vi "NLEIS_Run_PXI.vi"(0 "# of Amplitudes\n(Auto)":i32=5, 1 "Largest Amplitude (mA or mV)":dbl=0.01 format="%#.5f", 2 "Smallest Amplitude (mA or mV)":dbl=0.005 format="%#.6f", 4 "Steps/Decade":dbl=10.0, 5 "High Frequency (Hz)":dbl=10000.0, 6 "Internal Resistor":string(combo), 7 "Low Frequency (Hz)":dbl=1.0, 8 "Overload Action":string(combo)="OL0", 9 "File Path to Save":path=path "C:/Users/Giang/Desktop/NLEIS_test/test/1", 10 "Perturbation Input Gain":string(combo)="PI1", 11 "Amplitude Scaling File Location":path=path "C:/Users/Giang/Desktop/scaling_factors.txt", 12 "Voltage Output Gain":string(combo)="VX0", 14 "Current Output Gain":string(combo)="IX0") -> ()   [LabVIEW 2018]
doc: "This example shows the Standard Function output mode. \n\nIt also shows some of the parameters which can be changed on the fly."
uses:
  <vilib>/Utility/file.llb/Read From Spreadsheet File (DBL).vi
  <vilib>/Utility/file.llb/Write To Spreadsheet File (string).vi
panel:
  out "Error code 2":dbl
  out "Error code 1":dbl caption="Potentiostat \nError code 1"
  in  "Graph Tabs":enum32{"Active Run", "Nyquist Plot"}(tab)
  out "Avg Voltage FFT":cluster{"f0":dbl, "df":dbl, "magnitude":dbl[]}(graph)
  out "Avg Current FFT":cluster{"f0":dbl, "df":dbl, "magnitude":dbl[]}(graph)
  out "Avg I & V (Scaled)":waveform(dbl)[](graph) caption="Waveform \nGraph 3"
  in  "V Scale":dbl(slide) min=-6.0 max=0.0 step=1.0 scale=0.0..-6.0
  in  "I Scale":dbl(slide)=-3.0 min=-6.0 max=0.0 step=1.0 scale=0.0..-6.0
  out "Nyquist Plot":cluster{"Y":dbl[], "Y":dbl[]}[](graph)
  out "Actual End Time":timestamp format="%<%I:%M:%S %p\n%x>T"
  in  "NLEIS Run Mode":bool caption="Test        Sweep"
  in  "Bottom Tabs":enum32{"Status", "Generated Arrays"}(tab)
  out "Estimated End Time":timestamp format="%<%I:%M:%S %p\n%x>T"
  out "# Freqs":i32
  out "Actual Frequency":dbl format="%.6f"
  out "Freq Index":i32
  out "IR In Use":string
  out "FGEN Amp (V)":dbl
  out "Digitizer Loop\nComplete":bool
  out "Amp Index":i32
  out "# Amps":i32
  out "Cut-off Exceeded":bool
  out "Solartron Error":bool
  out "fp":dbl[](array[numeric]) format="%#.8f"
  out "Scaling Factors":sgl[](array[numeric])
  out "Amplitudes":dbl[](array[numeric])
  out "DAQ Error":string
  out "FGen Error":string caption="FGEN Error"
  out "DAQ Input":waveform(dbl)[](graph) caption="Waveform \nGraph 3"
  out "Pre-Check Voltage":dbl[](graph)
  in  "Middle Tabs":T1(tab)
  in  "Bandwidth":string(combo)="2"
  in  "Operation Mode":bool=TRUE
  in  "EIS File":bool
  in  "Time Files":bool=TRUE
  in  "Potentiostat":refnum<visa-resource-name>="Solartron1287"
  in  "FGen":refnum<k15>="FGEN-5421" caption="Waveform Generator"
  in  "NISCOPE":refnum<k15>="NISCOPE-5922" caption="Oscilloscope"
  in  "BiasReject ON?":bool
  in  "# Pre-Checks (>1Hz)":i32=10
  in  "Fixed Voltage Rejection (VRF)":string="VR0"
  in  "Fixed Current Rejection (IRF)":string="IR0"
  in  "Pre-Check Cut-Off (V)":dbl=0.5
  in  "# Pre-Checks (<1Hz)":i32=1
  in  "Direct Bias":string="PC0" caption="PCF (Amps)\nPVF (Volts)"
  in  "Bias Reject Mode":bool
  in  "Channel 1 (Voltage)":dbl=2.0
  in  "Channel 0 (Current)":dbl=2.0
  in  "Top Tabs":enum32{"Test", "Sweep", "Adv. Setup"}(tab)
  in  "Test Amplitude (mA or mV)":dbl=0.005
  in  "Peak Frequency (Hz)":dbl=5.0
  out "Too Many?":bool
  in  "Sweep Direction":bool
  in  "Crossover Freqs":string
  in  "Variable Resistor":bool
  in  "Manual # of Averages":i32=1
  in  "Signal Averages Selection":bool
  in  "# of Amps\n(Manual)":i32
  in  "Amplitude\nArray Source":bool
  in  "Manual Amplitudes":dbl[](array[numeric])
  # "Raw Digitizer Inputs"
  # "Pre-Check Voltage (Potentiostat)"
  # "Average Current and Voltage"
  # "Average Current Harmonics (FFT)"
  # "Average Voltage Harmonics (FFT)"
  # "Sweep Details"
  # "Active Run"
  # "Electrochemical Interface (SI1287) Setup"
  # "Write Files"
  # "Electrochemical Interface (SI1287) Setup"
  # "Bias Settings"
  # "Signal Precheck"
  # "Electrochemical Interface (SI1287) Setup"
  # "PStat Gain Control"
  # "PXI-5922 has two vertical range: \n1) 2 Vpk-pk, -1 -> +1 V\n2) 10 vpk-pk, -5 -> +5V"
  # "Vertical Range"
  # "Harmonic Tests Setup"
  # "Frequency Sweep Setup"
  # "Perturbation Amplitude Sweep (Auto)"
  # "Signal Processing Averaging Setup"
  # "Perturbation Amplitude Sweep (Manual)"
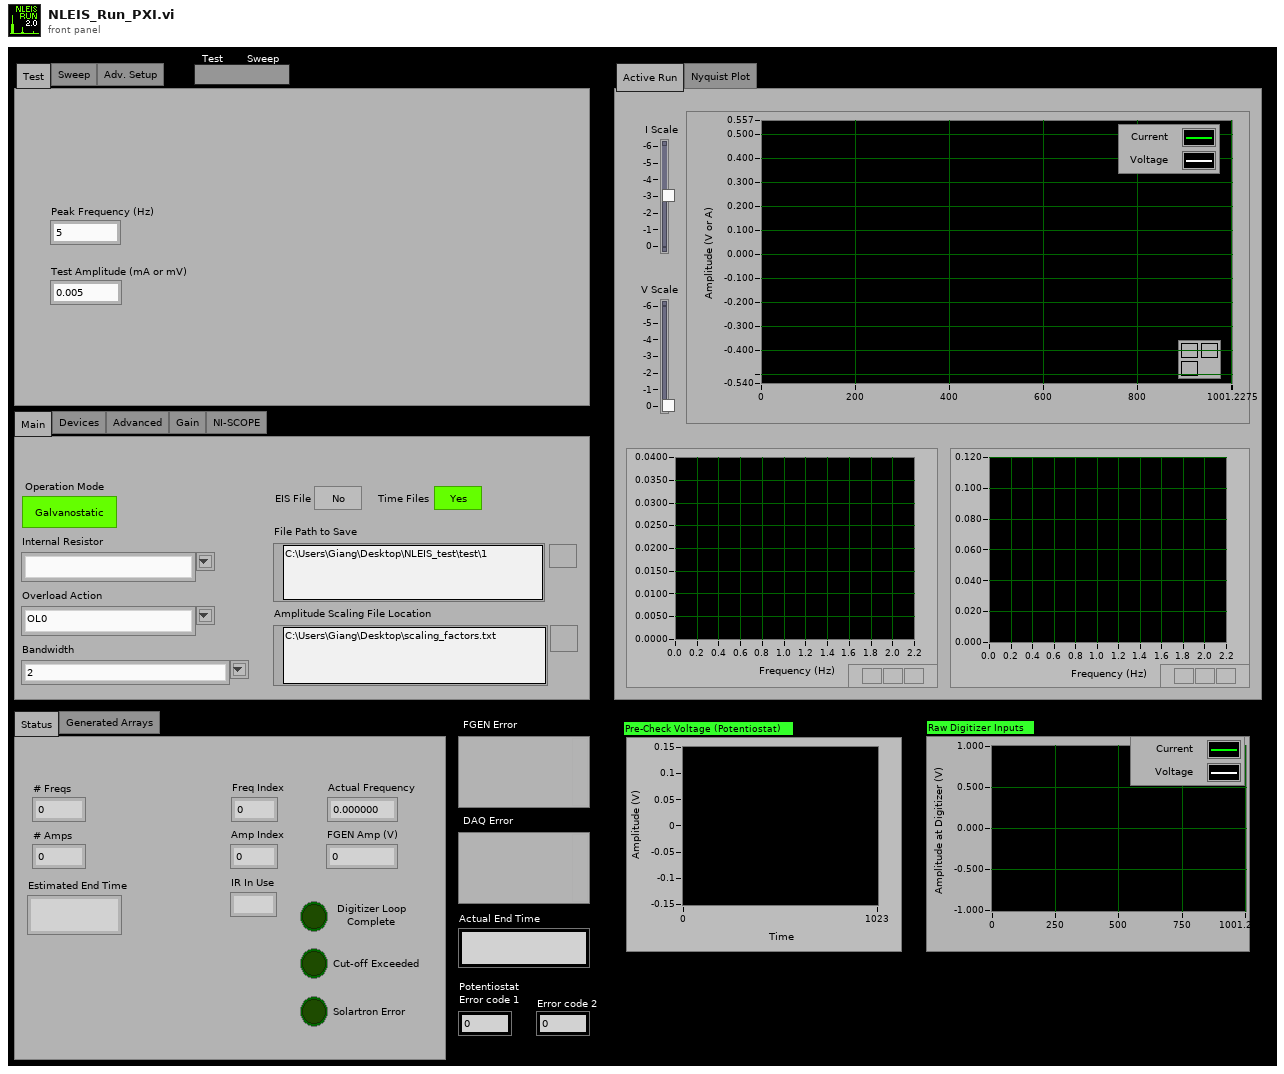
[diagram p1: front panel]
types:
  T1 = enum32{"Main", "Devices", "Advanced", "Gain", "NI-SCOPE"}
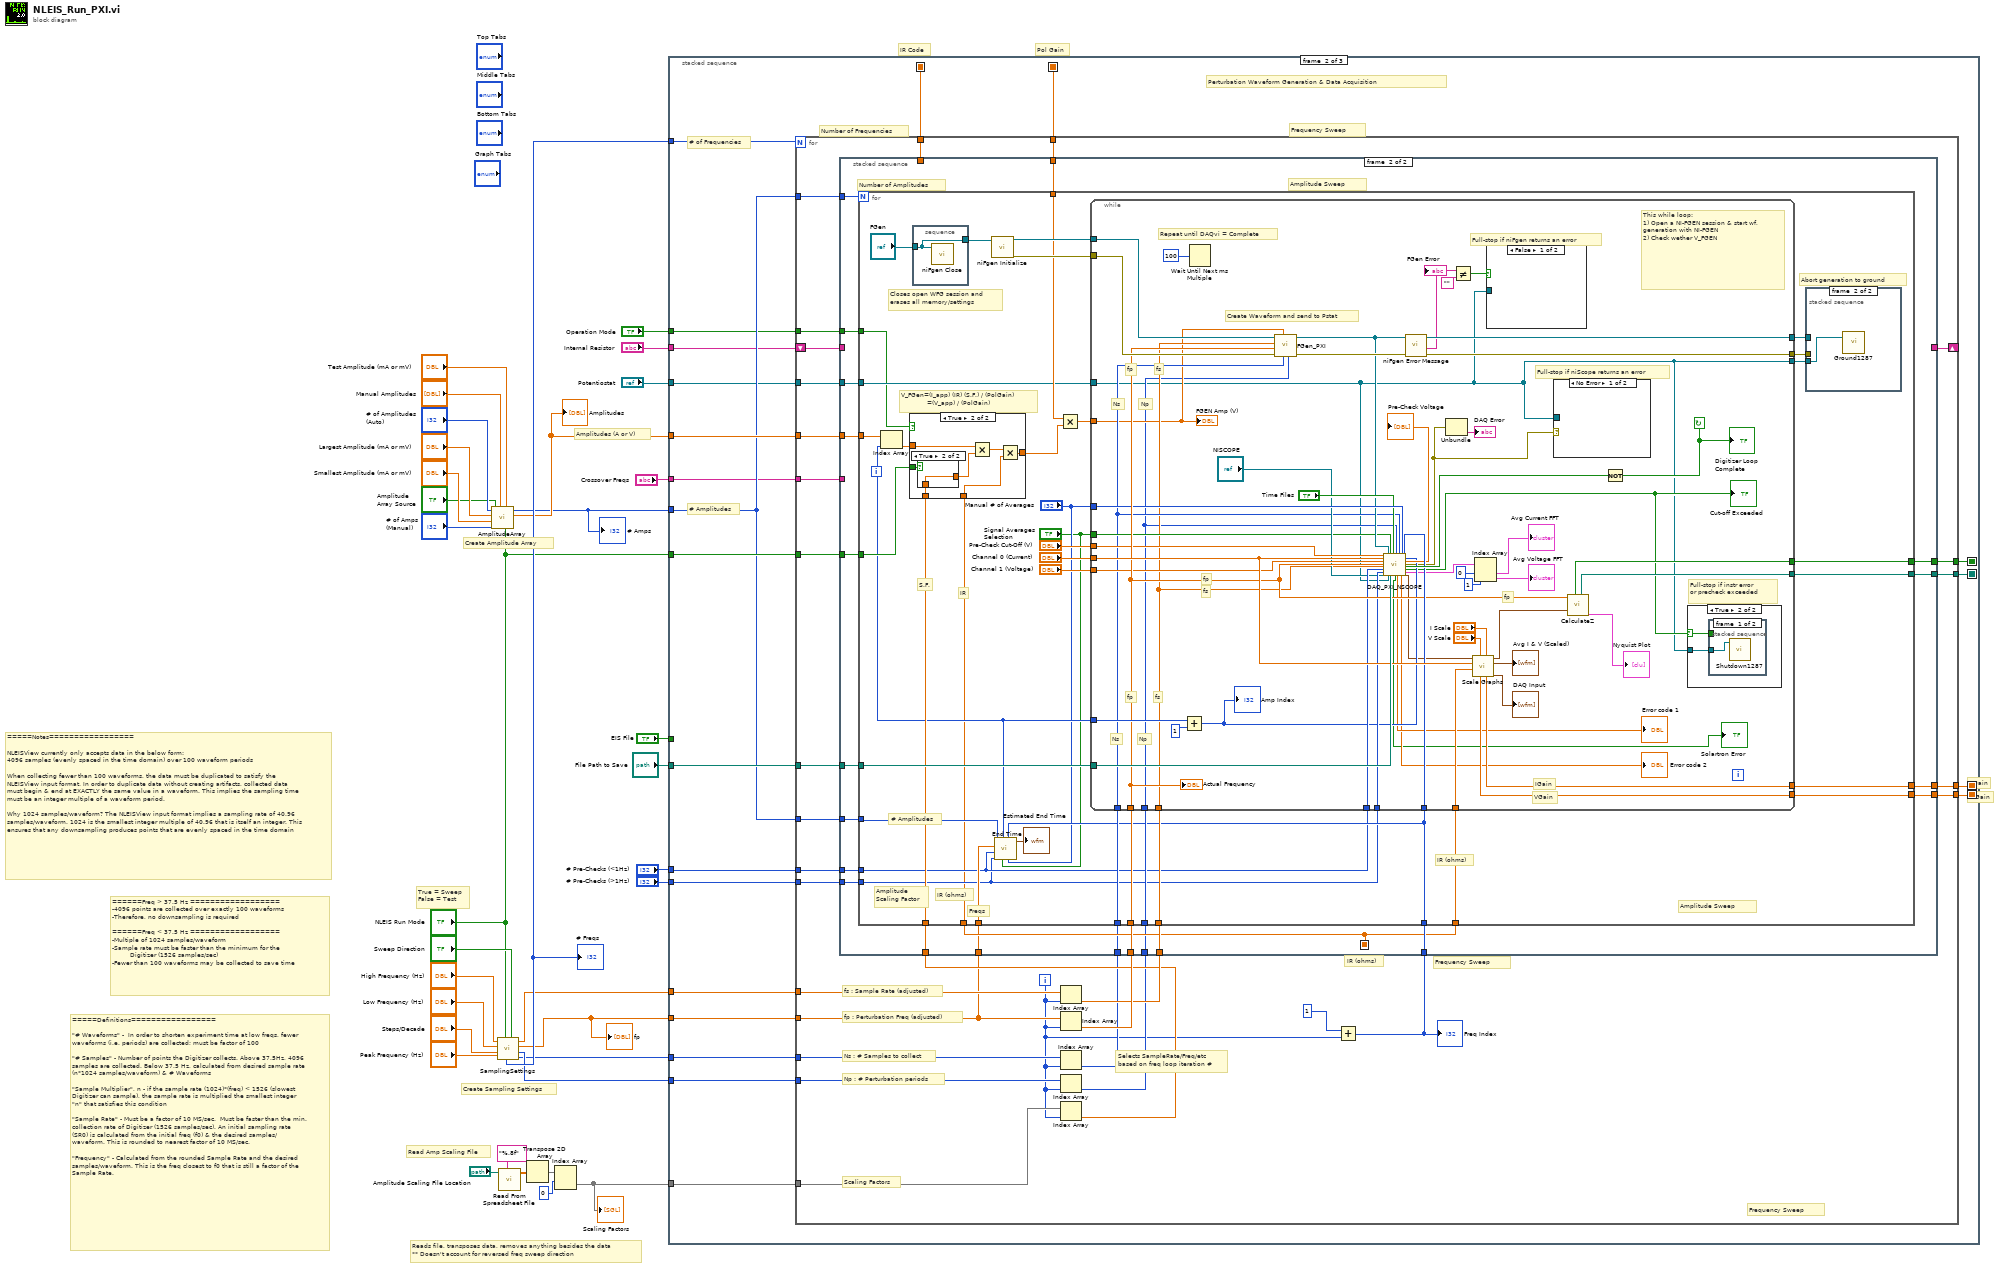
[diagram p0: block diagram]
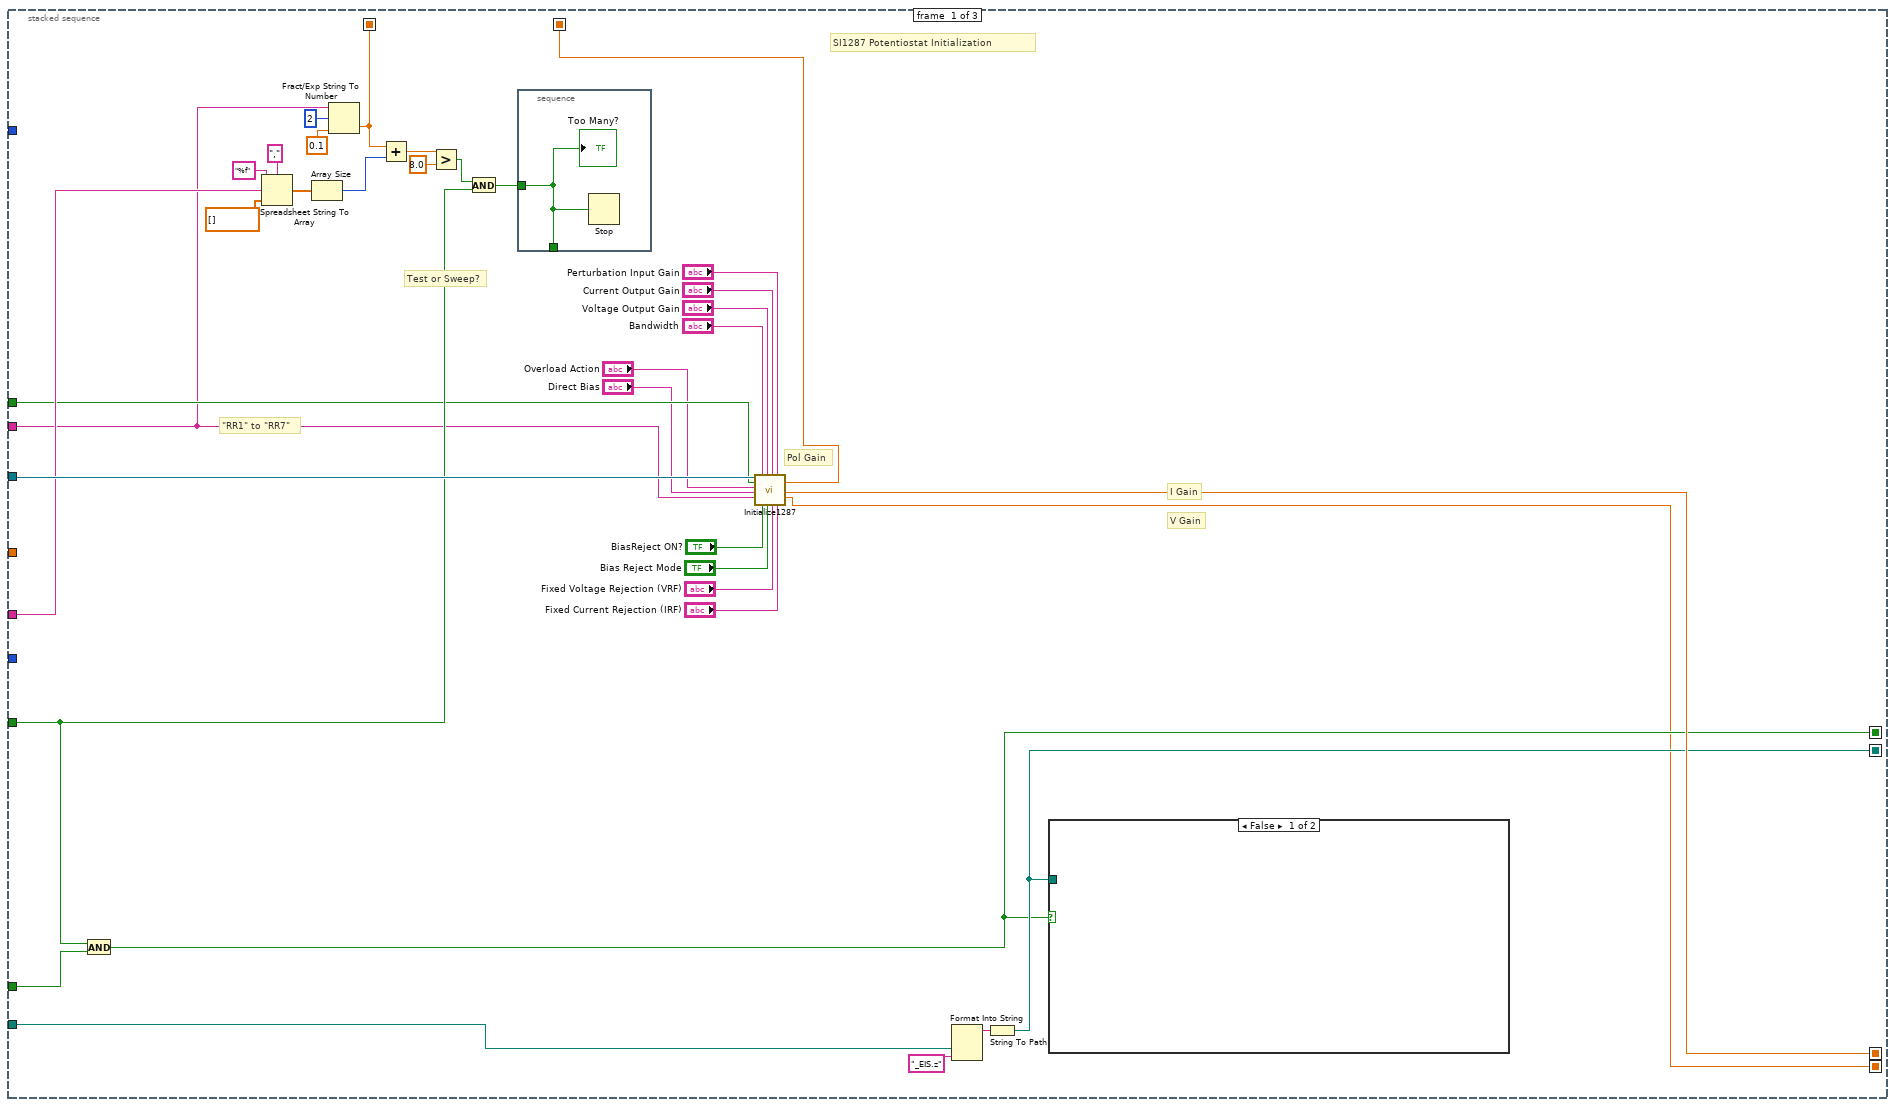
[diagram p2: hidden frame]
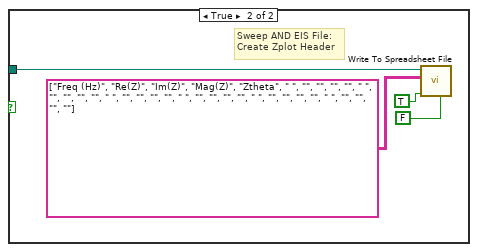
[diagram p3: hidden frame]
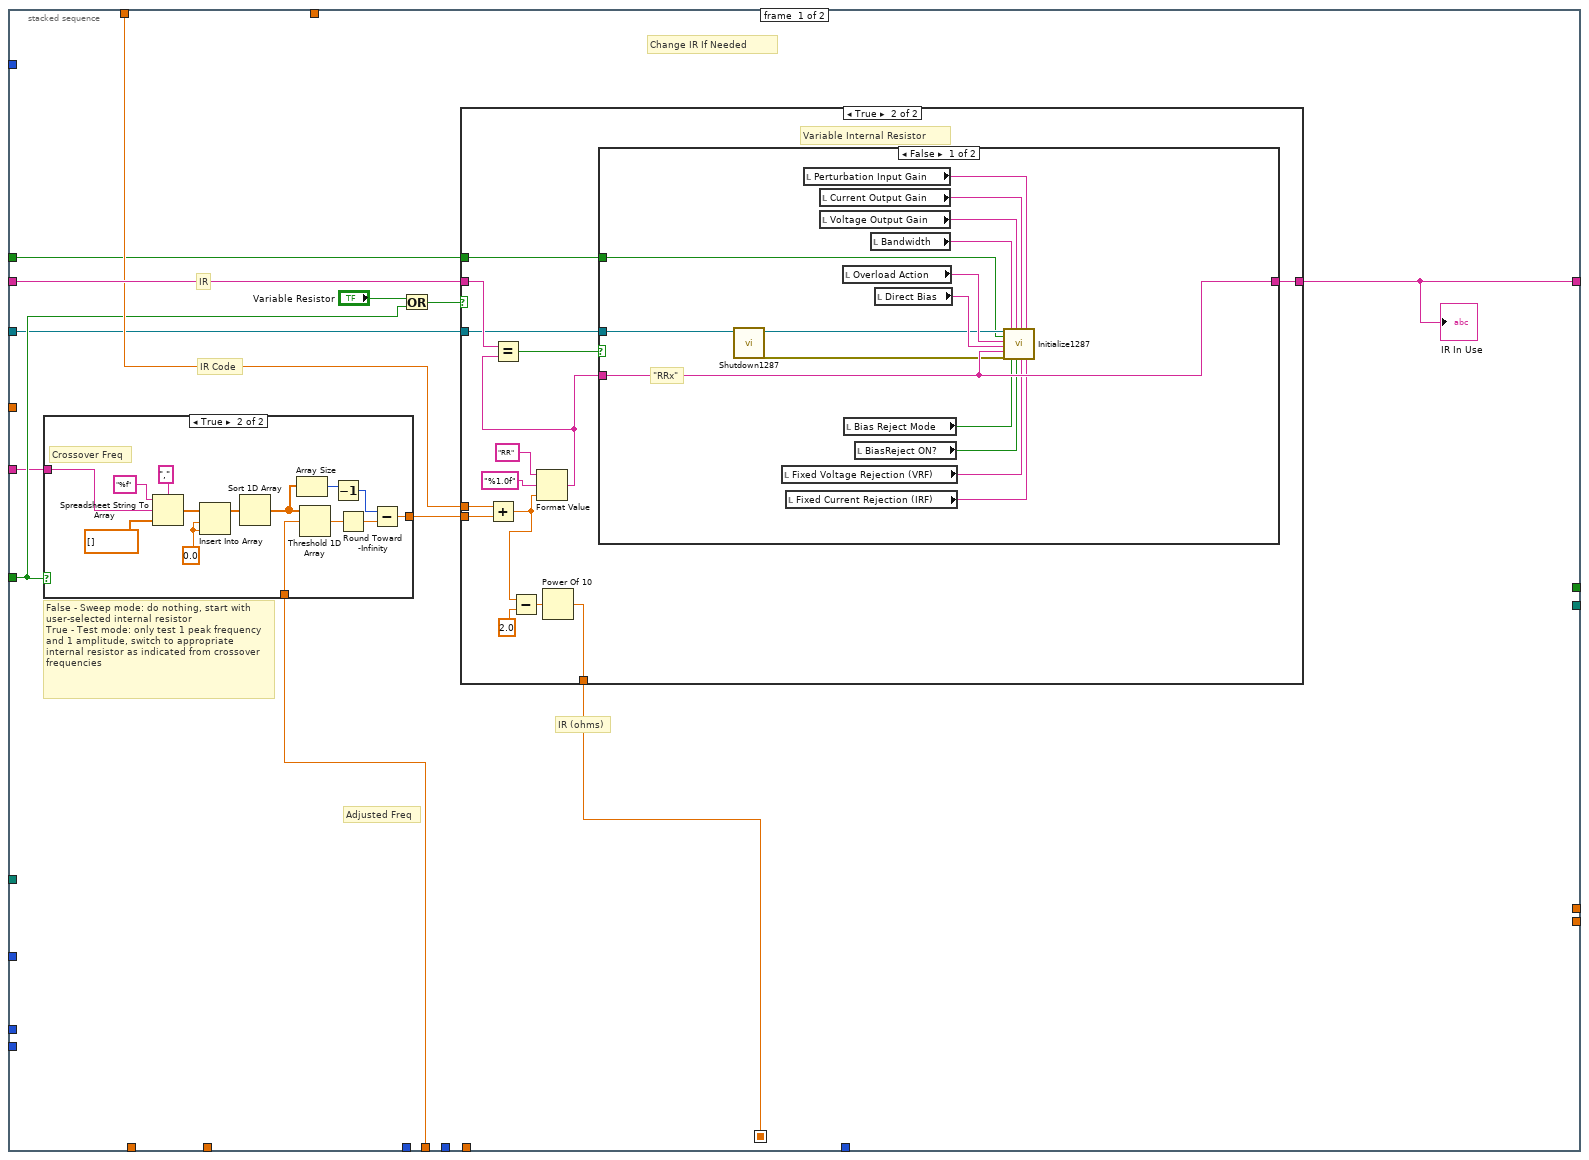
[diagram p4: hidden frame]
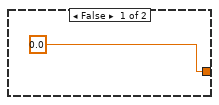
[diagram p5: hidden frame]
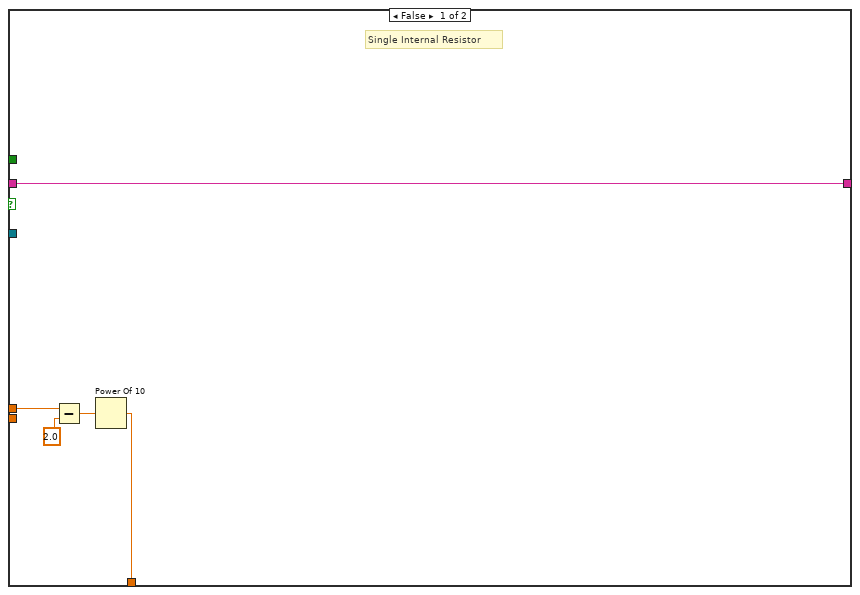
[diagram p6: hidden frame]
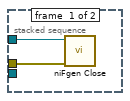
[diagram p8: hidden frame]
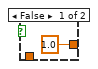
[diagram p10: hidden frame]
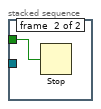
[diagram p12: hidden frame]
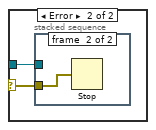
[diagram p13: hidden frame]
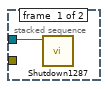
[diagram p14: hidden frame]
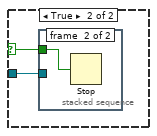
[diagram p15: hidden frame]
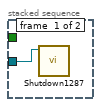
[diagram p16: hidden frame]
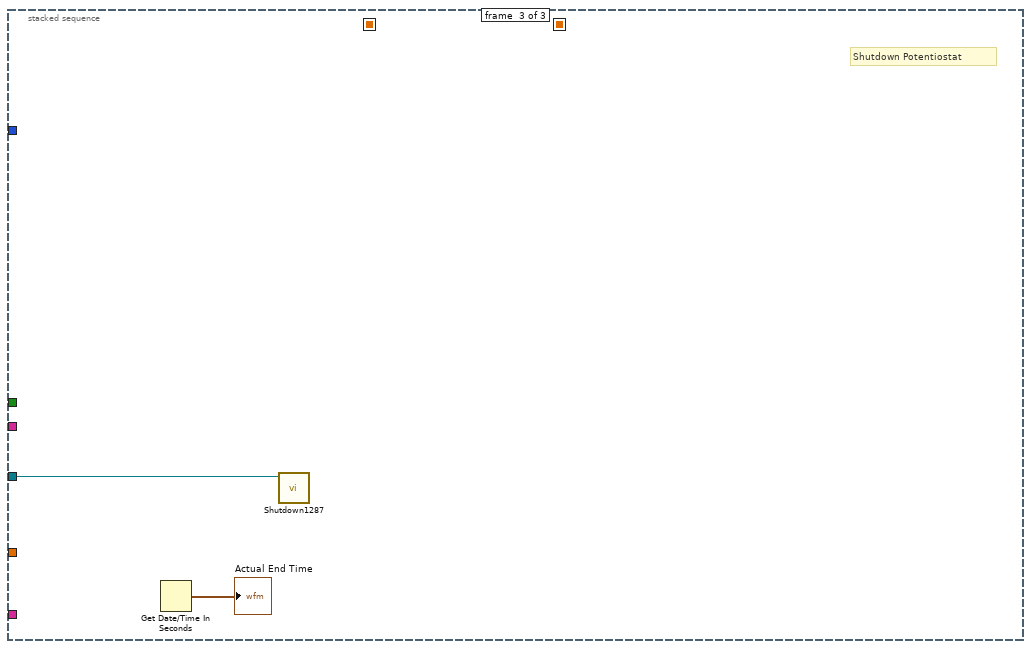
[diagram p17: hidden frame]
diagram:
  # "Amplitudes (A or V)"
  # "True = Sweep\nFalse = Test"
  # "Read Amp Scaling File"
  # "Reads file, transposes data, removes anything besides the data\n** Doesn't account for reversed freq sweep direction"
  # "V Gain"
  # "I Gain"
  # "IR Code"
  # "Pol Gain"
  # "Create Sampling Settings"
  # "Create Amplitude Array"
  # "=====Notes=================\n\nNLEISView currently only accepts data in the below form:\n4096 samples (evenly spaced in the time domain) over 100 waveform periods\n\nWhen collecting fewer than 100 waveforms, the data must be duplicated to satisfy the NLEISView input format. In order to duplicate data without creating artifacts, collected data must begin & end at EXACTLY the same value in a waveform. This implies the sampling time must be an integer multiple of a waveform period.\n\nWhy 1024 samples/waveform? The NLEISView input format implies a sampling rate of 40.96 samples/waveform. 1024 is the smallest integer multiple of 40.96 that is itself an integer. This ensures that any downsampling produces points that are evenly spaced in the time domain"
  # "=====Definitions=================\n\n\"# Waveforms\" -  In order to shorten experiment time at low freqs, fewer waveforms (i.e. periods) are collected; must be factor of 100\n\n\"# Samples\" - Number of points the Digitizer collects. Above 37.5Hz, 4096 samples are collected. Below 37.5 Hz, calculated from desired sample rate (n*1024 samples/waveform) & # Waveforms\n\n\"Sample Multiplier\", n - if the sample rate (1024)*(freq) < 1526 (slowest Digitizer can sample), the sample rate is multiplied the smallest integer \"n\" that satisfies this condition\n\n\"Sample Rate\" - Must be a factor of 10 MS/sec.  Must be faster than the min. collection rate of Digitizer (1526 samples/sec). An initial sampling rate (SR0) is calculated from the initial freq (f0) & the desired samples/waveform. This is rounded to nearest factor of 10 MS/sec.\n\n\"Frequency\" - Calculated from the rounded Sample Rate and the desired samples/waveform. This is the freq closest to f0 that is still a factor of the Sample Rate."
  # "======Freq > 37.5 Hz ==================\n-4096 points are collected over exactly 100 waveforms\n-Therefore, no downsampling is required\n\n======Freq < 37.5 Hz ==================\n-Multiple of 1024 samples/waveform\n-Sample rate must be faster than the minimum for the \n         Digitizer (1526 samples/sec)\n-Fewer than 100 waveforms may be collected to save time"
  n1 = call "AmplitudeArray.vi"("NLEIS Run Mode"="NLEIS Run Mode", "Test Amplitude (mA)"="Test Amplitude (mA or mV)", "Amplitude\nArray Source"="Amplitude\nArray Source", "Manual Amplitudes"="Manual Amplitudes", "# Amplitudes (Manual)"="# of Amps\n(Manual)", "Smallest Amplitude (mA)"="Smallest Amplitude (mA or mV)", "Largest Amplitude (mA)"="Largest Amplitude (mA or mV)", "# Amplitudes (Auto)"="# of Amplitudes\n(Auto)") -> ("Amplitudes (A)"=w17:dbl[], "# Amplitudes"=w4:i32)  [unwired: 2 in]
  "Amplitudes" <- w17
  "# Amps" <- w4
  n2 = call "SamplingSettings.vi"("Sweep Direction"="Sweep Direction", "NLEIS Run Mode"="NLEIS Run Mode", "Peak Frequency (Hz)"="Peak Frequency (Hz)", "Steps/Decade"="Steps/Decade", "Low Frequency (Hz)"="Low Frequency (Hz)", "High Frequency (Hz)"="High Frequency (Hz)") -> ("N Samples"=w25:i32[], "Np Periods"=w26:i32[], "Freqs"=w9:dbl[], "Sample Rates"=w27:dbl[], "Number of Frequencies"=w28:i32)  [unwired: 1 out]
  "# Freqs" <- w28
  "fp" <- w9
  n3 = call-poly <vilib>:"Read From Spreadsheet File.vi"("format (%.3f)"="%.8f", "file path (dialog if empty)"="Amplitude Scaling File Location") -> ("all rows"=w12:dbl[][])  [unwired: 5 in, 4 out]
  n4 = Transpose 2D Array(2D array=w12) -> (transposed array=w11:dbl[][])
  n5 = Index Array(array=w11, index (row)=0) -> (element=w10:dbl[])  [unwired: 1 in]
  "Scaling Factors" <- w10
  n6 = stacked-sequence {
    seq-local: [w62 _ _] -> [_ w93 _]
    seq-local: [w36 _ _] -> [_ w92 _]
    seq-local: [w35 _ _] -> [_ w91 _]
    seq-local: [w57 _ _] -> [_ w90 _]
    seq-local: [w52 _ _] -> [_ w79 _]
    seq-local: [w49 _ _] -> [_ w78 _]
    tunnel: "File Path to Save" -> [w53 w97 _]
    tunnel: w28 -> [_ w96 _]
    tunnel: w9 -> [_ w95 _]
    tunnel: w27 -> [_ w94 _]
    tunnel: "NLEIS Run Mode" -> [w50 w87 _]
    tunnel: w25 -> [_ w89 _]
    tunnel: w26 -> [_ w88 _]
    tunnel: w17 -> [_ w86 _]
    tunnel: w4 -> [_ w85 _]
    tunnel: w10 -> [_ w84 _]
    tunnel: "# Pre-Checks (<1Hz)" -> [_ w83 _]
    tunnel: "# Pre-Checks (>1Hz)" -> [_ w82 _]
    tunnel: "Potentiostat" -> [w58 w81 w334]
    tunnel: "Crossover Freqs" -> [w56 w80 _]
    tunnel: "EIS File" -> [w51 _ _]
    tunnel: "Operation Mode" -> [w44 w76 _]
    tunnel: "Internal Resistor" -> [w41 w77 _]
    frame #0 {
      # "\"RR1\" to \"RR7\""
      # "I Gain"
      # "V Gain"
      # "Pol Gain"
      # "Test or Sweep?"
      # "SI1287 Potentiostat Initialization"
      n7 = And(x=w50, y=w51) -> (x .and. y?=w49:bool)
      n8 = Spreadsheet String To Array(delimiter (Tab)=",", format string="%f", spreadsheet string=w56, array type (2D Dbl)=dbl[] []) -> (array=w61:dbl[])
      n9 = Array Size(array=w61) -> (size(s)=w65:i32)
      n10 = Fract/Exp String To Number(string=w41, offset=2, default (0 dbl)=0.1) -> (number=w62:dbl)  [unwired: 1 in, 1 out]
      n11 = Add(x=w62, y=w65) -> (x+y=w64:dbl)
      n12 = Greater?(x=w64, y=8.0) -> (0:w60:bool)
      n13 = And(x=w60, y=w50) -> (x .and. y?=w59:bool)
      n14 = stacked-sequence {
        tunnel: [w75] -> _
        tunnel: w59 -> [w75]
        frame #0 {
          n15 = Stop(stop? (T)=w75) -> ()
          "Too Many?" <- w75
        }
      }
      n16 = call "Initialize1287.vi"("VISA Name In"=w58, "Operation Mode"=w44, "Overload Action"="Overload Action", "DC Bias"="Direct Bias", "Internal Resistor"=w41, "Bandwidth"="Bandwidth", "Bias Rejection ON?"="BiasReject ON?", "Voltage Gain"="Voltage Output Gain", "Bias Reject Mode"="Bias Reject Mode", "Current Gain"="Current Output Gain", "Fixed Voltage Rejection"="Fixed Voltage Rejection (VRF)", "Perturbation Waveform Gain"="Perturbation Input Gain", "Fixed Current Rejection"="Fixed Current Rejection (IRF)") -> ("Pol Gain Correction"=w36:dbl, "I Gain Correction"=w57:dbl, "V Gain Correction"=w35:dbl)  [unwired: 2 in, 2 out]
      n17 = Format Into String(w53, "_EIS.z") -> (resulting string=w55:string)  [unwired: 3 in, 1 out]
      n18 = String To Path(string=w55) -> (path=w52:path)
      n19 = case shown="False" w49 {
        tunnel: w52 -> [_ w71]
        frame False {
        }
        frame True {
          # "Sweep AND EIS File:\nCreate Zplot Header"
          n20 = call-poly <vilib>:"Write To Spreadsheet File.vi"("transpose? (no:F)"=FALSE ("append to file? (new file:F)"), "append to file? (new file:F)"=TRUE, "2D data"=string[][] [["Freq (Hz)", "Re(Z)", "Im(Z)", "Mag(Z)", "Ztheta"], [" ", "", "", "", ""], [" ", "", "", "", ""], [" ", "", "", "", ""], [" ", "", "", "", ""], [" ", "", "", "", ""], [" ", "", "", "", ""]], "file path (dialog if empty)"=w71) -> ()  [unwired: 4 in, 1 out]
        }
      }
    }
    frame #1 {
      # "# of Frequencies"
      # "# Amplitudes"
      # "Frequency Sweep"
      # "Number of Frequencies"
      # "Perturbation Waveform Generation & Data Acquisition"
      n21 = for {
        N: w96 -> [_]
        tunnel: w97 -> [w128]
        tunnel: w95 -> [w112]
        tunnel: w94 -> [w124]
        tunnel: w86 -> [w127]
        tunnel: w85 -> [w126]
        shift-right: [w119] -> _
        shift-left: w77 -> [w118]
        tunnel: w93 -> [w117]
        tunnel: w87 -> [w116]
        tunnel: w92 -> [w115]
        tunnel: w91 -> [w114]
        tunnel: w90 -> [w113]
        tunnel: w85 -> [w111]
        tunnel: w89 -> [w110]
        tunnel: w88 -> [w109]
        tunnel: w84 -> [w106]
        tunnel: w83 -> [w105]
        tunnel: w82 -> [w104]
        tunnel: w81 -> [w103]
        tunnel: w80 -> [w102]
        tunnel: w78 -> [w101]
        tunnel: w79 -> [w100]
        tunnel: w76 -> [w99]
        i -> [w98]
        # "Frequency Sweep"
        # "IR (ohms)"
        # "Scaling Factors"
        # "Np : # Perturbation periods"
        # "Ns : # Samples to collect"
        # "fp : Perturbation Freq (adjusted)"
        # "fs : Sample Rate (adjusted)"
        # "Frequency Sweep"
        # "Selects SampleRate/Freq/etc\nbased on freq loop iteration #"
        n22 = Index Array(array=w124, index=w98) -> (element=w122:dbl)
        n23 = Index Array(array=w112, index=w98) -> (element=w123:dbl)
        n24 = Index Array(array=w110, index=w98) -> (element=w108:i32)
        n25 = Index Array(array=w109, index=w98) -> (element=w107:i32)
        n26 = Index Array(array=w106, index=w98) -> (element=w120:dbl)
        n27 = Add(x=1, y=w98) -> (x+y=w121:i32)
        "Freq Index" <- w121
        n28 = stacked-sequence {
          seq-local: [w139 _] -> [_ w204]
          tunnel: w128 -> [_ w212]
          tunnel: w127 -> [_ w211]
          tunnel: w126 -> [_ w210]
          tunnel: w123 -> [w138 w209]
          tunnel: w122 -> [_ w208]
          tunnel: w121 -> [_ w207]
          tunnel: w120 -> [_ w206]
          tunnel: [w140 _] -> w119
          tunnel: w118 -> [w137 _]
          tunnel: w117 -> [w135 _]
          tunnel: w116 -> [w133 w205]
          tunnel: w115 -> [_ w203]
          tunnel: w114 -> [_ w202]
          tunnel: w113 -> [_ w201]
          tunnel: w112 -> [_ w200]
          tunnel: w111 -> [_ w199]
          tunnel: w108 -> [_ w198]
          tunnel: w107 -> [_ w197]
          tunnel: w105 -> [_ w196]
          tunnel: w104 -> [_ w195]
          tunnel: w103 -> [w131 w194]
          tunnel: w102 -> [w130 _]
          tunnel: w101 -> [_ w193]
          tunnel: w100 -> [_ w192]
          tunnel: w99 -> [w129 w191]
          frame #0 {
            # "False - Sweep mode: do nothing, start with user-selected internal resistor\nTrue - Test mode: only test 1 peak frequency and 1 amplitude, switch to appropriate internal resistor as indicated from crossover frequencies"
            # "IR (ohms)"
            # "IR Code"
            # "IR"
            # "Change IR If Needed"
            # "Adjusted Freq"
            n29 = case shown="True" w133 {
              tunnel: w138 -> [_ w147]
              tunnel: [0.0 w146] -> w136
              tunnel: w130 -> [_ w142]
              frame False {
              }
              frame True {
                w143 = 0.0
                # "Crossover Freq"
                n30 = Spreadsheet String To Array(delimiter (Tab)=",", format string="%f", spreadsheet string=w142, array type (2D Dbl)=dbl[] []) -> (array=w145:dbl[])
                n31 = Insert Into Array(array=w145, index=w143, new element=w143) -> (w144:dbl[])
                n32 = Sort 1D Array(array=w144) -> (sorted array=w152:dbl[])
                n33 = Array Size(array=w152) -> (size(s)=w149:i32)
                n34 = Threshold 1D Array(2:w147, 3:w152) -> (0:w151:dbl)  [unwired: 1 in]
                n35 = Decrement(x=w149) -> (x-1=w148:i32)
                n36 = Round Toward -Infinity(1:w151) -> (0:w150:dbl)
                n37 = Subtract(x=w148, y=w150) -> (x-y=w146:dbl)
              }
            }
            n38 = Or(x="Variable Resistor", y=w133) -> (x .or. y?=w132:bool)
            n39 = case shown="True" w132 {
              tunnel: [w159 w174] -> w140
              tunnel: w137 -> [w159 w173]
              tunnel: [w160 w167] -> w139
              tunnel: w136 -> [_ w169]
              tunnel: w135 -> [w157 w168]
              tunnel: w131 -> [_ w162]
              tunnel: w129 -> [_ w161]
              frame False {
                # "Single Internal Resistor"
                n40 = Subtract(x=w157, y=2.0) -> (x-y=w156:dbl)
                n41 = Power Of 10(x=w156) -> (10^x=w160:dbl)
              }
              frame True {
                # "Variable Internal Resistor"
                n42 = Add(x=w168, y=w169) -> (x+y=w164:dbl)
                n43 = Subtract(x=w164, y=2.0) -> (x-y=w163:dbl)
                n44 = Format Value(string ("")="RR", format string="%1.0f", value (0)=w164) -> (output string=w166:string)
                n45 = Equal?(x=w173, y=w166) -> (x = y?=w172:bool)
                n46 = Power Of 10(x=w163) -> (10^x=w167:dbl)
                n47 = case shown="False" w172 {
                  tunnel: w166 -> [w189 w190]
                  tunnel: [w189 w190] -> w174
                  tunnel: w162 -> [w185 _]
                  tunnel: w161 -> [w182 _]
                  frame False {
                    # "\"RRx\""
                    n48 = call "Shutdown1287.vi"("VISA Name In"=w185) -> ("error out"=w183:errorcluster, "VISA resource name out"=w184:refnum<visa-resource-name>)  [unwired: 7 in]
                    n49 = local read "Fixed Voltage Rejection (VRF)"() -> (w177:string)
                    n50 = local read "Fixed Current Rejection (IRF)"() -> (w176:string)
                    n51 = local read "Perturbation Input Gain"() -> (w175:string)
                    n52 = local read "Current Output Gain"() -> (w181:string)
                    n53 = local read "Voltage Output Gain"() -> (w180:string)
                    n54 = local read "Overload Action"() -> (w188:string)
                    n55 = local read "Bias Reject Mode"() -> (w179:bool)
                    n56 = local read "BiasReject ON?"() -> (w178:bool)
                    n57 = local read "Bandwidth"() -> (w187:string)
                    n58 = local read "Direct Bias"() -> (w186:string)
                    n59 = call "Initialize1287.vi"("VISA Name In"=w184, "Operation Mode"=w182, "Overload Action"=w188, "DC Bias"=w186, "Internal Resistor"=w189, "Error In (No Error)"=w183, "Bandwidth"=w187, "Bias Rejection ON?"=w179, "Voltage Gain"=w180, "Bias Reject Mode"=w178, "Current Gain"=w181, "Fixed Voltage Rejection"=w177, "Perturbation Waveform Gain"=w175, "Fixed Current Rejection"=w176) -> ()  [unwired: 1 in, 5 out]
                  }
                  frame True {
                  }
                }
              }
            }
            "IR In Use" <- w140
          }
          frame #1 {
            # "Amplitude Sweep"
            # "Number of Amplitudes"
            n60 = for {
              N: w210 -> [_]
              tunnel: w209 -> [w232]
              tunnel: w212 -> [w251]
              tunnel: w206 -> [w240]
              tunnel: w208 -> [w245]
              tunnel: w207 -> [w225]
              tunnel: w211 -> [w244]
              tunnel: w204 -> [w215]
              tunnel: w205 -> [w241]
              tunnel: w204 -> [w236]
              tunnel: w203 -> [w235]
              tunnel: w202 -> [w234]
              tunnel: w201 -> [w233]
              tunnel: w200 -> [w229]
              tunnel: w199 -> [w227]
              tunnel: w198 -> [w231]
              tunnel: w197 -> [w230]
              tunnel: w196 -> [w224]
              tunnel: w195 -> [w223]
              tunnel: w194 -> [w220]
              tunnel: w193 -> [w218]
              tunnel: w192 -> [w217]
              tunnel: w191 -> [w214]
              i -> [w226]
              # "Abort generation to ground"
              # "IR"
              # "IR (ohms)"
              # "S.F."
              # "IR (ohms)"
              # "# Amplitudes"
              # "Amplitude Sweep"
              # "Freqs"
              # "Amplitude\nScaling Factor"
              # "Closes open WFG session and \nerases all memory/settings"
              # "V_FGen=(I_app) (IR) (S.F.) / (PolGain)\n             =(V_app) / (PolGain)"
              n61 = Index Array(array=w244, index=w226) -> (element=w216:dbl)
              n62 = case shown="True" w214 {
                tunnel: w241 -> [_ w261]
                tunnel: w240 -> [_ w260]
                tunnel: [w255 w259] -> w239
                tunnel: w216 -> [w255 w258]
                tunnel: w215 -> [_ w256]
                frame False {
                }
                frame True {
                  n63 = case shown="True" w261 {
                    tunnel: w260 -> [_ w264]
                    tunnel: [1.0 w264] -> w257
                    frame False {
                    }
                    frame True {
                    }
                  }
                  n64 = Multiply(x=w258, y=w257) -> (x*y=w262:dbl)
                  n65 = Multiply(x=w262, y=w256) -> (x*y=w259:dbl)
                }
              }
              n66 = stacked-sequence {
                tunnel: [w265] -> w248
                tunnel: "FGen" -> [w265]
                frame #0 {
                  n67 = call <instrlib>:"niFgen Close.vi"("Instrument Handle"=w265) -> ()  [unwired: 10 in, 1 out]
                }
              }
              n68 = call <instrlib>:"niFgen Initialize.vi"("Resource Name"=w248) -> ("error out"=w246:errorcluster, "Instrument Handle Out"=w247:refnum<k15>)  [unwired: 9 in]
              n69 = call "End Time.vi"("Manual # of Averages"="Manual # of Averages", "Freq Index"=w225, "Signal Averages Selection"="Signal Averages Selection", "Amp Index"=w226, "# of Pre-Check Points Collected (above 1 HZ)"=w223, "Np to Pre-Check (<1Hz)"=w224, "fp Array"=w229, "# Amplitudes"=w227) -> ("Estimated \nEnd Time"=→"Estimated End Time":timestamp)  [unwired: 3 in]
              n70 = Multiply(x=w235, y=w239) -> (x*y=w238:dbl)
              n71 = while {
                tunnel: w246 -> [w316]
                tunnel: [w320] -> w249
                tunnel: [w321] -> w250
                tunnel: w232 -> [w311]
                tunnel: w238 -> [w272]
                tunnel: w251 -> [w318]
                tunnel: w226 -> [w317]
                tunnel: w247 -> [w315]
                tunnel: "Channel 0 (Current)" -> [w313]
                tunnel: "Channel 1 (Voltage)" -> [w277]
                tunnel: w245 -> [w273]
                tunnel: w225 -> [w312]
                tunnel: "Pre-Check Cut-Off (V)" -> [w310]
                tunnel: w236 -> [w309]
                tunnel: w234 -> [w308]
                tunnel: w233 -> [w307]
                tunnel: w224 -> [w306]
                tunnel: w223 -> [w305]
                tunnel: w231 -> [w274]
                tunnel: w230 -> [w271]
                tunnel: "Signal Averages Selection" -> [w275]
                tunnel: "Manual # of Averages" -> [w304]
                tunnel: w220 -> [w267]
                tunnel: w218 -> [w303]
                tunnel: w217 -> [w302]
                tunnel: [w267] -> w213
                stop <- w314 continue-if-true
                # "Full-stop if instr error \nor precheck exceeded"
                # "Full-stop if niScope returns an error"
                # "Full-stop if niFgen returns an error"
                # "Np"
                # "Ns"
                # "fp"
                # "fs"
                # "fp"
                # "fs"
                # "fp"
                # "Np"
                # "Ns"
                # "fp"
                # "fs"
                # "Repeat until DAQvi = Complete"
                # "Create Waveform and send to Pstat"
                # "This while loop:\n1) Open a NI-FGEN session & start wf, generation with NI-FGEN\n2) Check wether V_FGEN"
                # "IGain"
                # "VGain"
                n72 = Add(x=w317, y=1) -> (x+y=w292:i32)
                "Amp Index" <- w292
                n73 = Wait Until Next ms Multiple(millisecond multiple=u32 100) -> ()  [unwired: 1 out]
                n74 = call "FGen_PXI.vi"("Np"=w271, "Ns"=w274, "FGen Amplitude (V)"=w272, "error in (no error)"=w316, "fp (wfm)"=w311, "fs (input)"=w273, "Instrument Handle"=w315) -> ("error out"=w295:errorcluster, "Instrument Handle Out"=w279:refnum<k15>)  [unwired: 3 in]
                n75 = call "DAQ_PXI_NSCOPE.vi"("Pre-Check Cut-Off (V)"=w310, "Range Ch0 (A)"=w313, "Range Ch1 (V)"=w277, "Frequency (fp)"=w311, "Sample Rate (fs)"=w273, "# Pre-Checks <1Hz"=w306, "# Pre-Checks >1Hz"=w305, "Oscilloscope"="NISCOPE", "FGen Handle"=w279, "Potentiostat"=w267, "Auto/Manual \nSignal Averaging"=w275, "file path (dialog if empty)"=w318, "Write Time Data"="Time Files", "# Periods (Np)"=w271, "# Samples (Ns)"=w274, "Manual # Signal Avgs"=w304, "Frequency Run #"=w312, "Amplitude Run #"=w292) -> ("Solartron Error"=→"Solartron Error":bool, "Error code 1"=→"Error code 1":dbl, "Error code 2"=→"Error code 2":dbl, "Pre-Check Voltage"=→"Pre-Check Voltage":dbl[], "DAQ Error"=w278:errorcluster, "Measurement Complete"=w319:bool, "Cut-Off Exceeded"=w268:bool, "Avg Data (FFT)"=w286:cluster{"f0":dbl, "df":dbl, "magnitude":dbl[]}[], "Avg Data"=w285:waveform(dbl)[])  [unwired: 1 in]
                "Cut-off Exceeded" <- w268
                n76 = call <instrlib>:"niFgen Error Message.vi"("error in (no error)"=w295, "Instrument Handle"=w279) -> ("error out"=w320:errorcluster, "Error Message"=w299:string, "Instrument Handle Out"=w321:refnum<k15>)  [unwired: 6 in, 1 out]
                "FGen Error" <- w299
                n77 = Unbundle(w278) -> ("source"=→"DAQ Error":string)  [unwired: 2 out]
                n78 = Not Equal?(x=w299, y="") -> (x != y?=w298:bool)
                n79 = call "Scale Graphs.vi"("IGain"=w307, "I Scale"="I Scale", "VGain"=w308, "V Scale"="V Scale", "IR (ohms)"=w309, "Channel 0 (Current)"=w313, "Wfm Data"=w285) -> ("DAQ Input"=→"DAQ Input":waveform(dbl)[], "Scaled Wfm (I,V)"=→"Avg I & V (Scaled)":waveform(dbl)[], "Wfm (I,V)"=w282:waveform(dbl)[])  [unwired: 2 in]
                n80 = Index Array(array=w286, index #1=0 ("index"), index #2=1 ("index")) -> (element #1=→"Avg Current FFT":cluster{"f0":dbl, "df":dbl, "magnitude":dbl[]}, element #2=→"Avg Voltage FFT":cluster{"f0":dbl, "df":dbl, "magnitude":dbl[]})
                n81 = case shown="False" w298 {
                  selector: w298 -> [_ w331]
                  tunnel: w267 -> [_ w330]
                  frame False {
                  }
                  frame True {
                    n82 = stacked-sequence {
                      tunnel: w331 -> [_ w333]
                      tunnel: w330 -> [w332 _]
                      frame #0 {
                        n83 = call "Shutdown1287.vi"("VISA Name In"=w332) -> ()  [unwired: 7 in, 2 out]
                      }
                      frame #1 {
                        n84 = Stop(stop? (T)=w333) -> ()
                      }
                    }
                  }
                }
                n85 = case shown="No Error" w278 {
                  selector: w278 -> [_ w327]
                  tunnel: w267 -> [_ w326]
                  frame No Error {
                  }
                  frame Error {
                    n86 = stacked-sequence {
                      tunnel: w327 -> [_ w329]
                      tunnel: w326 -> [w328 _]
                      frame #0 {
                        n87 = call "Shutdown1287.vi"("VISA Name In"=w328) -> ()  [unwired: 7 in, 2 out]
                      }
                      frame #1 {
                        n88 = Stop(stop? (T)=w329) -> ()
                      }
                    }
                  }
                }
                n89 = call "CalculateZ.vi"("File Path to Save"=w302, "EIS File"=w303, "Avg I & V"=w282, "Frequency"=w311) -> ("Nyquist Plot"=→"Nyquist Plot":cluster{"Y":dbl[], "Y":dbl[]}[])  [unwired: 2 in, 5 out]
                n90 = Not(x=w319) -> (.not. x?=w314:bool)
                "Digitizer Loop\nComplete" <- w314
                n91 = case shown="True" w268 {
                  selector: w268 -> [_ w323]
                  tunnel: w267 -> [_ w322]
                  frame False {
                  }
                  frame True {
                    n92 = stacked-sequence {
                      tunnel: w323 -> [_ w325]
                      tunnel: w322 -> [w324 _]
                      frame #0 {
                        n93 = call "Shutdown1287.vi"("VISA Name In"=w324) -> ()  [unwired: 7 in, 2 out]
                      }
                      frame #1 {
                        n94 = Stop(stop? (T)=w325) -> ()
                      }
                    }
                  }
                }
                "Actual Frequency" <- w311
                "FGEN Amp (V)" <- w272
              }
              n95 = stacked-sequence {
                tunnel: w250 -> [w253 _]
                tunnel: w249 -> [w252 _]
                tunnel: w213 -> [_ w254]
                frame #0 {
                  n96 = call <instrlib>:"niFgen Close.vi"("error in (no error)"=w252, "Instrument Handle"=w253) -> ()  [unwired: 9 in, 1 out]
                }
                frame #1 {
                  n97 = call "Ground1287.vi"("VISA Name In"=w254) -> ()  [unwired: 1 in, 2 out]
                }
              }
            }
          }
        }
      }
    }
    frame #2 {
      # "Shutdown Potentiostat"
      n98 = Get Date/Time In Seconds() -> (seconds since 1Jan1904=→"Actual End Time":timestamp)
      n99 = call "Shutdown1287.vi"("VISA Name In"=w334) -> ()  [unwired: 7 in, 2 out]
    }
  }
